vi "PCO_Recording.vi"() -> (0 "PCO_Recording":T1, 1 "PCO_Recording_Raw":T2, 2 "Length":u16, 3 "Raw_Length":u16)   [LabVIEW 2019, in "SDK.lvlib" / "Structures.lvlib"]
doc: "Use this template to build a VI to use as a subVI."
uses:
  Structures.lvlib
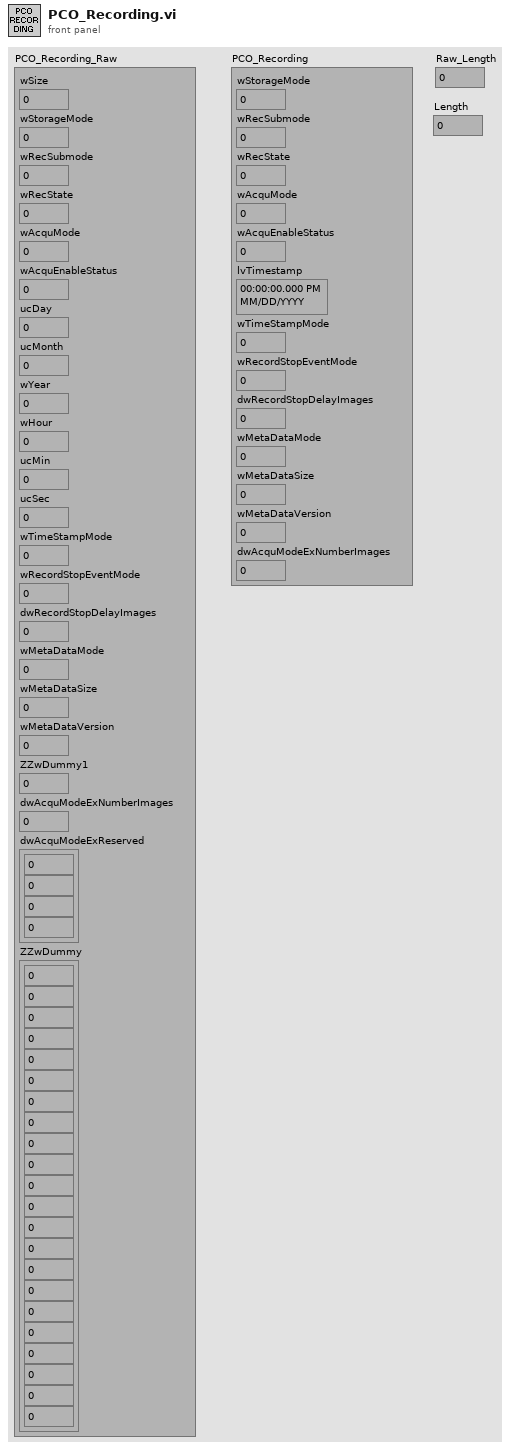
[diagram p1: front panel]
types:
  T1 = cluster{"wStorageMode":u16, "wRecSubmode":u16, "wRecState":u16, "wAcquMode":u16, "wAcquEnableStatus":u16, "lvTimestamp":timestamp, "wTimeStampMode":u16, "wRecordStopEventMode":u16, "dwRecordStopDelayImages":u32, "wMetaDataMode":u16, "wMetaDataSize":u16, "wMetaDataVersion":u16, "dwAcquModeExNumberImages":u32}
  T2 = cluster{"wSize":u16, "wStorageMode":u16, "wRecSubmode":u16, "wRecState":u16, "wAcquMode":u16, "wAcquEnableStatus":u16, "ucDay":u8, "ucMonth":u8, "wYear":u16, "wHour":u16, "ucMin":u8, "ucSec":u8, "wTimeStampMode":u16, "wRecordStopEventMode":u16, "dwRecordStopDelayImages":u32, "wMetaDataMode":u16, "wMetaDataSize":u16, "wMetaDataVersion":u16, "ZZwDummy1":u16, "dwAcquModeExNumberImages":u32, "dwAcquModeExReserved":cluster{u32, u32, u32, u32}, "ZZwDummy":cluster{u16, u16, u16, u16, u16, u16, u16, u16, u16, u16, u16, u16, u16, u16, u16, u16, u16, u16, u16, u16, u16, u16}}
  T3 = cluster{u16, u16, u16, u16, u16, u16, u16, u16, u16, u16, u16, u16, u16, u16, u16, u16, u16, u16, u16, u16, u16, u16}
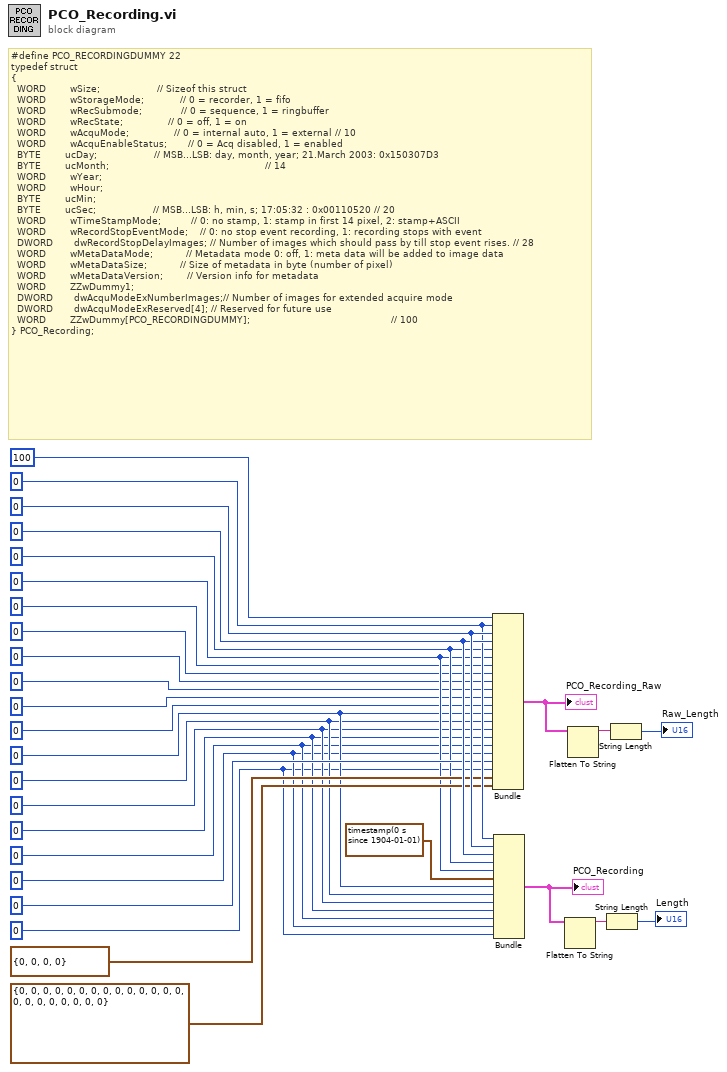
[diagram p0: block diagram]
diagram:
  w3 = u32 0 ("dwAcquModeExNumberImages")
  w4 = u16 0 ("wMetaDataVersion")
  w5 = u16 0 ("wMetaDataSize")
  w6 = u16 0 ("wMetaDataMode")
  w7 = u32 0 ("dwRecordStopDelayImages")
  w8 = u16 0 ("wRecordStopEventMode")
  w9 = u16 0 ("wTimeStampMode")
  w16 = u16 0 ("wAcquEnableStatus")
  w17 = u16 0 ("wAcquMode")
  w22 = u16 0 ("wRecState")
  w23 = u16 0 ("wRecSubmode")
  w21 = u16 0 ("wStorageMode")
  # "#define PCO_RECORDINGDUMMY 22\ntypedef struct\n{\n  WORD        wSize;                   // Sizeof this struct\n  WORD        wStorageMode;            // 0 = recorder, 1 = fifo\n  WORD        wRecSubmode;             // 0 = sequence, 1 = ringbuffer\n  WORD        wRecState;               // 0 = off, 1 = on\n  WORD        wAcquMode;               // 0 = internal auto, 1 = external // 10\n  WORD        wAcquEnableStatus;       // 0 = Acq disabled, 1 = enabled\n  BYTE        ucDay;                   // MSB...LSB: day, month, year; 21.March 2003: 0x150307D3\n  BYTE        ucMonth;                                                    // 14\n  WORD        wYear;\n  WORD        wHour;\n  BYTE        ucMin;\n  BYTE        ucSec;                   // MSB...LSB: h, min, s; 17:05:32 : 0x00110520 // 20\n  WORD        wTimeStampMode;          // 0: no stamp, 1: stamp in first 14 pixel, 2: stamp+ASCII\n  WORD        wRecordStopEventMode;    // 0: no stop event recording, 1: recording stops with event\n  DWORD       dwRecordStopDelayImages; // Number of images which should pass by till stop event rises. // 28\n  WORD        wMetaDataMode;           // Metadata mode 0: off, 1: meta data will be added to image data\n  WORD        wMetaDataSize;           // Size of metadata in byte (number of pixel)\n  WORD        wMetaDataVersion;        // Version info for metadata\n  WORD        ZZwDummy1;\n  DWORD       dwAcquModeExNumberImages;// Number of images for extended acquire mode\n  DWORD       dwAcquModeExReserved[4]; // Reserved for future use\n  WORD        ZZwDummy[PCO_RECORDINGDUMMY];                                               // 100\n} PCO_Recording;"
  n1 = Bundle("wSize"=u16 100, "wStorageMode"=w21, "wRecSubmode"=w23, "wRecState"=w22, "wAcquMode"=w17, "wAcquEnableStatus"=w16, "ucDay"=u8 0, "ucMonth"=u8 0, "wYear"=u16 0, "wHour"=u16 0, "ucMin"=u8 0, "ucSec"=u8 0, "wTimeStampMode"=w9, "wRecordStopEventMode"=w8, "dwRecordStopDelayImages"=w7, "wMetaDataMode"=w6, "wMetaDataSize"=w5, "wMetaDataVersion"=w4, "ZZwDummy1"=u16 0, "dwAcquModeExNumberImages"=w3, "dwAcquModeExReserved"=cluster{u32, u32, u32, u32} {0, 0, 0, 0}, "ZZwDummy"=T3 {0, 0, 0, 0, 0, 0, 0, 0, 0, 0, 0, 0, 0, 0, 0, 0, 0, 0, 0, 0, 0, 0}) -> (w24:T2)  [unwired: 1 in]
  "PCO_Recording_Raw" <- w24
  n2 = Bundle("wStorageMode"=w21, "wRecSubmode"=w23, "wRecState"=w22, "wAcquMode"=w17, "wAcquEnableStatus"=w16, "lvTimestamp"=timestamp(0 s since 1904-01-01), "wTimeStampMode"=w9, "wRecordStopEventMode"=w8, "dwRecordStopDelayImages"=w7, "wMetaDataMode"=w6, "wMetaDataSize"=w5, "wMetaDataVersion"=w4, "dwAcquModeExNumberImages"=w3) -> (w2:T1)  [unwired: 1 in]
  "PCO_Recording" <- w2
  n3 = Flatten To String(anything=w2) -> (data string=w29:string)  [unwired: 3 in, 2 out]
  n4 = Flatten To String(anything=w24) -> (data string=w28:string)  [unwired: 3 in, 2 out]
  n5 = String Length(string=w29) -> (length=→"Length":i32)
  n6 = String Length(string=w28) -> (length=→"Raw_Length":i32)
